vi "MQTTSubClient.vi"() -> ()   [LabVIEW 2017]
uses:
  <vilib>/daq.io/MQTT LabVIEW Client/Controls/QoS.ctl
  <vilib>/daq.io/MQTT LabVIEW Client/MQTT_Functions.lvlib
panel:
  out "PingReq Message":u8[](array[numeric]) format="%x"
  in  "stop":bool
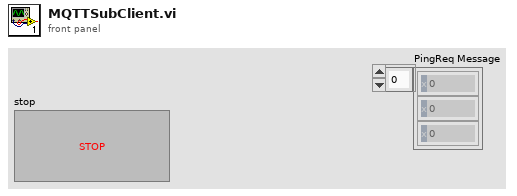
[diagram p1: front panel]
types:
  T1 = typedef "MQTT_Functions.lvlib/QoS.ctl" = enum8{"At most once", "At least once", "Exactly once", "Reserved"}
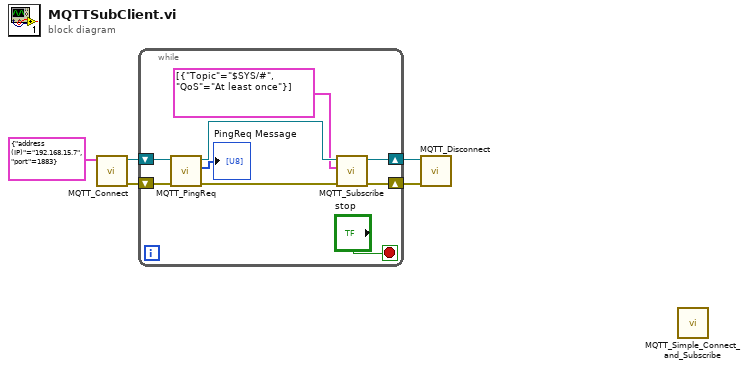
[diagram p0: block diagram]
diagram:
  n1 = call <vilib>:"MQTT_Connect.vi"("MQTT Broker"=cluster{"address (IP)":string, "port":u16} {"address (IP)"="192.168.15.7", "port"=1883}) -> ("error out"=w5:errorcluster, "connection ID out"=w4:refnum<k5>)  [unwired: 8 in, 1 out]
  n2 = while {
    shift-right: [w10] -> w3
    shift-left: w5 -> [w12]
    shift-right: [w9] -> w2
    shift-left: w4 -> [w11]
    stop <- "stop" stop-if-true
    n3 = call <vilib>:"MQTT_PingReq.vi"("error in (no error)"=w12, "connection ID"=w11) -> ("error out"=w14:errorcluster, "PingReq Message"=→"PingReq Message":u8[], "connection ID out"=w13:refnum<k5>)  [unwired: 7 in]
    n4 = call <vilib>:"MQTT_Subscribe.vi"("error in (no error)"=w14, "Subscription Info Array"=cluster{"Topic":string, "QoS":T1}[] [{"Topic"="$SYS/#", "QoS"=enum."At least once"}], "connection ID"=w13) -> ("error out"=w10:errorcluster, "connection ID out"=w9:refnum<k5>)  [unwired: 7 in]
  }
  n5 = call <vilib>:"MQTT_Disconnect.vi"("error in (no error)"=w3, "connection ID"=w2) -> ()  [unwired: 9 in, 1 out]
  n6 = call <vilib>:"MQTT_Simple_Connect_and_Subscribe.vi"() -> ()  [unwired: 12 in]
